vi "HE_state.vi"(6 "ZB":bool[](array[boolean])=[FALSE, FALSE], 7 "Alarm":bool[](array[boolean])=[FALSE, FALSE], 9 "XB":bool[](array[boolean])=[FALSE, FALSE, FALSE, FALSE, FALSE], 10 "Z_control":T5={"Z_HSw"=1, "Z_HSetState"=enum."on", "Z_ASetState"=enum."on", "Z_DSetState"=enum."on"}, 11 "HE1_state_in":refnum<class "HE_state.lvclass">) -> (1 "YB":bool[](array[boolean]), 2 "Z":T1={"Z_Source"=enum."local disabled", "Z_SetState"=enum."on", "Z_State"=enum."alarm", "Z_State_T"=0, "ZM_State"=enum."initialization", "ZM_State_T"=0, "ALR  L1"=FALSE, "ALR  L2"=FALSE, "HH_run"=0}, 3 "HE1_state_out":refnum<class "HE_state.lvclass">, 5 "ALR_ON":bool[](array[boolean]))   [LabVIEW 2019, in "Heating.lvlib" / "HE_state.lvclass"]
uses:
  HE_state.lvclass
  ctl/Z_control.ctl
  ctl/Z_State.ctl
  ctl/Z.ctl
  ctl/Z_source.ctl
  ctl/ZM_State.ctl
  HE_state.lvclass/HE_state.ctl
  ZM_state/HE_ZM_state.lvclass/HE_ZM_state.ctl
  Z_state/HE_Z_state.lvclass/HE_Z_state.ctl
  Sequence/State/State.lvclass/State.ctl
  Sequence/State/Read T (ms).vi
  Z_state/HE_Z_state.lvclass
  D:/my_projects/projects/Algorithms/Labview/19/Sequence/State/State.lvclass
  ZM_state/HE_ZM_state.lvclass
  Sequence/State/Step.vi
  Heating.lvlib
panel:
  # "Alarm_L1"
  # "Alarm_L2"
  # "Ki_XB01 contactor on"
  # "Ki_XB02 contactor off"
  # "XB24 local hand on"
  # "heating end"
  # "cooling end"
  # "Ki_ZB01 contactor on reg"
  # "Ki_ZB02 contactor off reg"
  # "TsStop"
  # "T_check"
  # "T_start_delay"
  # "T_heat_start"
  # "T_stop_delay"
  # "T_set_min"
  # "T_heat_stop"
  # "T_restart_delay"
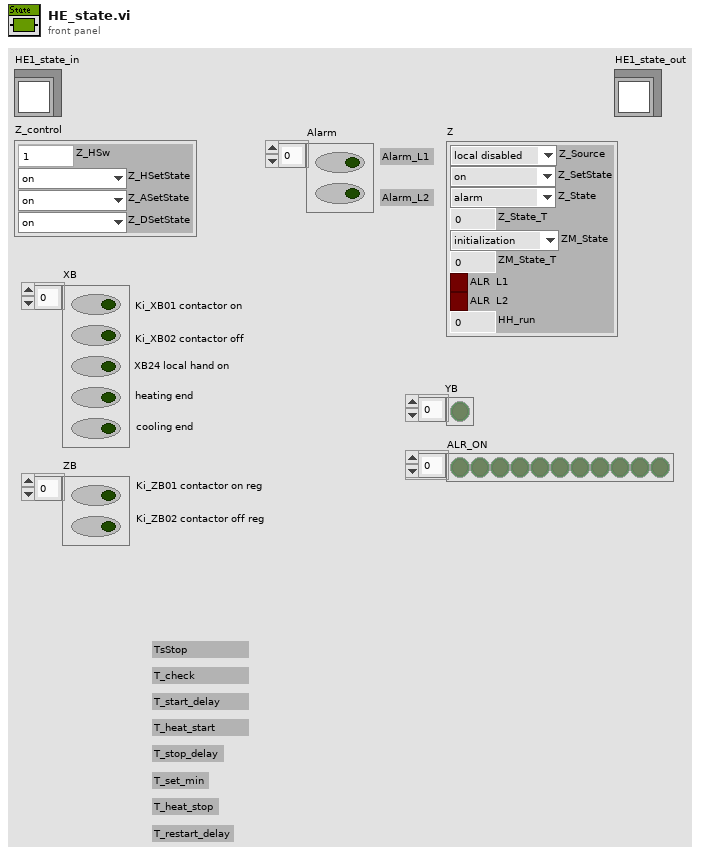
[diagram p1: front panel]
types:
  T1 = typedef "Heating.lvlib/Z.ctl" = cluster{"Z_Source":T2, "Z_SetState":T3, "Z_State":T3, "Z_State_T":u32, "ZM_State":T4, "ZM_State_T":u32, "ALR  L1":bool, "ALR  L2":bool, "HH_run":u64}
  T2 = typedef "Heating.lvlib/Z_source.ctl" = enum8{"initialize", "local disabled", "local hand", "hand", "auto", "dist"}
  T3 = typedef "Heating.lvlib/Z_State.ctl" = enum8{"initialization", "alarm", "disabled", "not ready", "stop ready", "reserv", "switched off", "reserv2", "switched on", "check", "on min", "decrease out", "on", "increase out", "on max"}
  T4 = typedef "Heating.lvlib/ZM_State.ctl" = enum8{"initialization", "stop", "start_cmd", "contactor_on_cmd", "heating", "on", "stop_cmd", "power_down", "contactor_off_cmd", "cooling", "restart_delay"}
  T5 = typedef "Heating.lvlib/Z_control.ctl" = cluster{"Z_HSw":u8, "Z_HSetState":T3, "Z_ASetState":T3, "Z_DSetState":T3}
  T6 = cluster{"Z_Source":T2, "Z_SetState":T3, "ZM_State":T4}
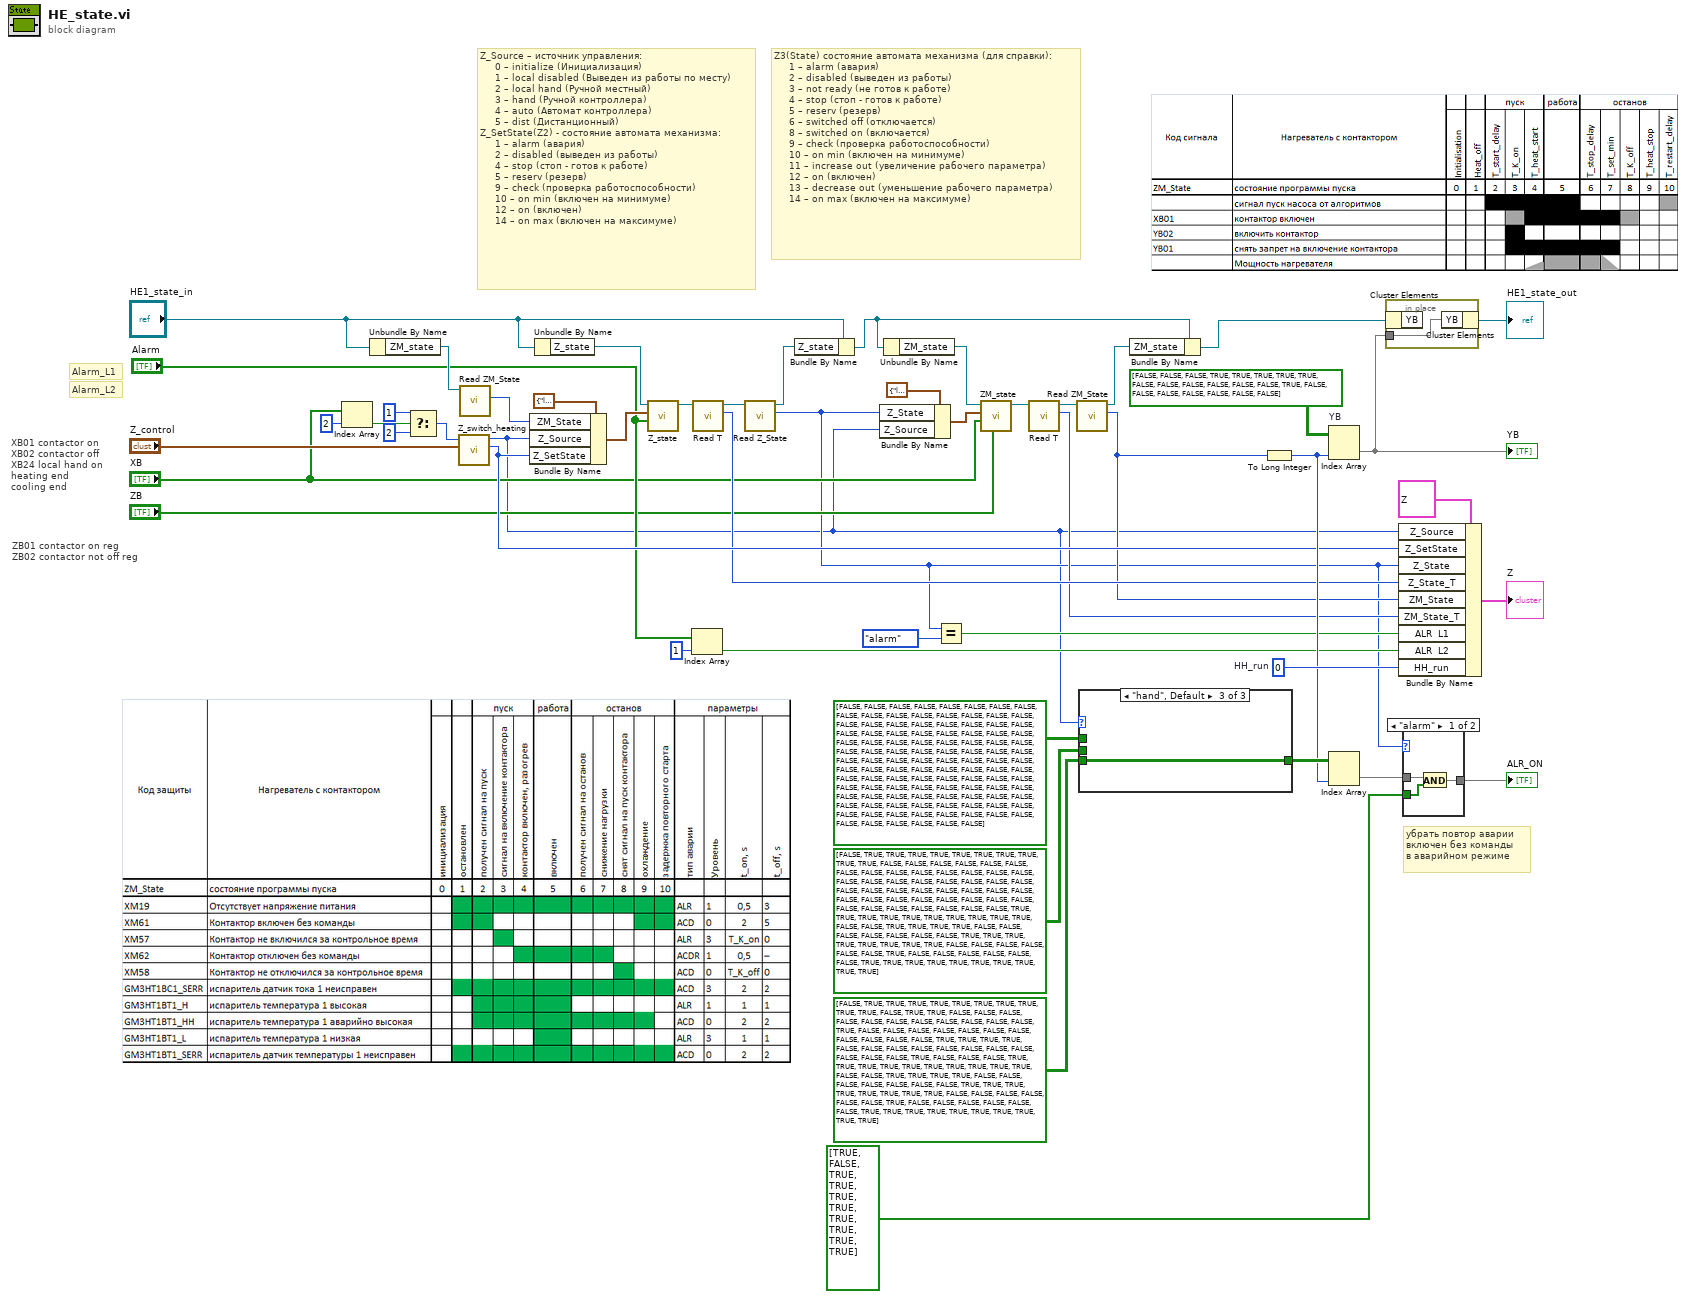
[diagram p0: block diagram]
diagram:
  w34 = 0  # HH_run
  # "Alarm_L2"
  # "Alarm_L1"
  # "ZB01 contactor on reg\nZB02 contactor not off reg"
  # "XB01 contactor on\nXB02 contactor off\nXB24 local hand on\nheating end\ncooling end"
  # "убрать повтор аварии\nвключен без команды\nв аварийном режиме"
  # "Z_Source – источник управления:\n     0 – initialize (Инициализация)\n     1 – local disabled (Выведен из работы по месту)\n     2 – local hand (Ручной местный)\n     3 – hand (Ручной контроллера)\n     4 – auto (Автомат контроллера)\n     5 – dist (Дистанционный)\nZ_SetState(Z2) - состояние автомата механизма:\n     1 – alarm (авария)\n     2 – disabled (выведен из работы)\n     4 – stop (стоп - готов к работе)\n     5 – reserv (резерв)\n     9 – check (проверка работоспособности)\n     10 – on min (включен на минимуме)\n     12 – on (включен)\n     14 – on max (включен на максимуме)"
  # "Z3(State) состояние автомата механизма (для справки):\n     1 – alarm (авария)\n     2 – disabled (выведен из работы)\n     3 – not ready (не готов к работе)\n     4 – stop (стоп - готов к работе)\n     5 – reserv (резерв)\n     6 – switched off (отключается)\n     8 – switched on (включается)\n     9 – check (проверка работоспособности)\n     10 – on min (включен на минимуме)\n     11 – increase out (увеличение рабочего параметра)\n     12 – on (включен)\n     13 – decrease out (уменьшение рабочего параметра)\n     14 – on max (включен на максимуме)"
  n1 = Index Array(array="XB", index=2) -> (element=w36:bool)
  n2 = Unbundle By Name("HE1_state_in") -> ("ZM_state"=w26:refnum<class "HE_ZM_state.lvclass">)
  n3 = Select(t=u8 1, s=w36, f=u8 2) -> (s? t:f=w44:u8)
  n4 = call "Z_switch_heating.vi"("Z"="Z_control", "Z_LSw"=w44) -> ("Z_SetState"=w27:T3, "Z_Source"=w6:T2)  [unwired: 8 in]
  n5 = call "Read ZM_State.vi"("HE_ZM_state in"=w26) -> ("ZM_State"=w25:T4)  [unwired: 9 in, 1 out]
  n6 = Bundle By Name(cluster=T6 {"Z_Source"=enum."local disabled", "Z_SetState"=enum."alarm", "ZM_State"=enum."initialization"} ("Z_In"), "ZM_State"=w25, "Z_Source"=w6, "Z_SetState"=w27) -> (w24:T6)
  n7 = Unbundle By Name("HE1_state_in") -> ("Z_state"=w23:refnum<class "HE_Z_state.lvclass">)
  n8 = call "Z_state.vi"("Alarm"="Alarm", "Z_In"=w24, "HE1_Z_state in"=w23) -> ("HE1_Z_state out"=w21:refnum<class "HE_Z_state.lvclass">)  [unwired: 8 in]
  n9 = Index Array(array="Alarm", index=1) -> (element=w29:bool)
  n10 = call "Read T.vi"("HE1_Z_state in"=w21) -> ("T (ms)"=w19:u32, "HE1_Z_state out"=w20:refnum<class "HE_Z_state.lvclass">)  [unwired: 9 in]
  n11 = call "Read Z_State.vi"("HE1_Z_state in"=w20) -> ("Z_State_heating"=w8:T3, "HE1_Z_state out"=w17:refnum<class "HE_Z_state.lvclass">)  [unwired: 9 in]
  n12 = Bundle By Name(cluster="HE1_state_in", "Z_state"=w17) -> (w4:refnum<class "HE_state.lvclass">)
  n13 = Bundle By Name(cluster=cluster{"Z_Source":T2, "Z_State":T3} {"Z_Source"=enum."local disabled", "Z_State"=enum."alarm"} ("Z_In"), "Z_State"=w8, "Z_Source"=w6) -> (w7:cluster{"Z_Source":T2, "Z_State":T3})
  n14 = Unbundle By Name(w4) -> ("ZM_state"=w16:refnum<class "HE_ZM_state.lvclass">)
  n15 = Equal?(x=w8, y=Z_State."alarm") -> (x = y?=w31:bool)
  n16 = call "ZM_state.vi"("ZB"="ZB", "XB"="XB", "Z_In"=w7, "ZM_state in"=w16) -> ("ZM_state out"=w15:refnum<class "HE_ZM_state.lvclass">)  [unwired: 7 in]
  n17 = call "Read T.vi"("valve_VCH_ZM_state in"=w15) -> ("T (ms)"=w12:u32, "valve_VCH_ZM_state out"=w14:refnum<class "HE_ZM_state.lvclass">)  [unwired: 9 in]
  n18 = call "Read ZM_State.vi"("HE_ZM_state in"=w14) -> ("ZM_State"=w13:T4, "HE_ZM_state out"=w5:refnum<class "HE_ZM_state.lvclass">)  [unwired: 9 in]
  n19 = case shown="\"hand\", Default" w6 {
    tunnel: bool[][] [[FALSE, FALSE, FALSE, FALSE, FALSE, FALSE, FALSE, FALSE, FALSE, FALSE, FALSE], [FALSE, FALSE, FALSE, FALSE, FALSE, FALSE, FALSE, FALSE, FALSE, FALSE, FALSE], [FALSE, FALSE, FALSE, FALSE, FALSE, FALSE, FALSE, FALSE, FALSE, FALSE, FALSE], [FALSE, FALSE, FALSE, FALSE, FALSE, FALSE, FALSE, FALSE, FALSE, FALSE, FALSE], [FALSE, FALSE, FALSE, FALSE, FALSE, FALSE, FALSE, FALSE, FALSE, FALSE, FALSE], [FALSE, FALSE, FALSE, FALSE, FALSE, FALSE, FALSE, FALSE, FALSE, FALSE, FALSE], [FALSE, FALSE, FALSE, FALSE, FALSE, FALSE, FALSE, FALSE, FALSE, FALSE, FALSE], [FALSE, FALSE, FALSE, FALSE, FALSE, FALSE, FALSE, FALSE, FALSE, FALSE, FALSE], [FALSE, FALSE, FALSE, FALSE, FALSE, FALSE, FALSE, FALSE, FALSE, FALSE, FALSE], [FALSE, FALSE, FALSE, FALSE, FALSE, FALSE, FALSE, FALSE, FALSE, FALSE, FALSE]] -> [w51 _ _]
    tunnel: bool[][] [[FALSE, TRUE, TRUE, TRUE, TRUE, TRUE, TRUE, TRUE, TRUE, TRUE, TRUE], [FALSE, FALSE, FALSE, FALSE, FALSE, FALSE, FALSE, FALSE, FALSE, FALSE, FALSE], [FALSE, FALSE, FALSE, FALSE, FALSE, FALSE, FALSE, FALSE, FALSE, FALSE, FALSE], [FALSE, FALSE, FALSE, FALSE, FALSE, FALSE, FALSE, FALSE, FALSE, FALSE, FALSE], [FALSE, FALSE, FALSE, FALSE, FALSE, FALSE, FALSE, FALSE, FALSE, FALSE, FALSE], [FALSE, TRUE, TRUE, TRUE, TRUE, TRUE, TRUE, TRUE, TRUE, TRUE, TRUE], [FALSE, FALSE, TRUE, TRUE, TRUE, TRUE, FALSE, FALSE, FALSE, FALSE, FALSE], [FALSE, FALSE, TRUE, TRUE, TRUE, TRUE, TRUE, TRUE, TRUE, TRUE, FALSE], [FALSE, FALSE, FALSE, FALSE, FALSE, TRUE, FALSE, FALSE, FALSE, FALSE, FALSE], [FALSE, TRUE, TRUE, TRUE, TRUE, TRUE, TRUE, TRUE, TRUE, TRUE, TRUE]] -> [_ w52 _]
    tunnel: bool[][] [[FALSE, TRUE, TRUE, TRUE, TRUE, TRUE, TRUE, TRUE, TRUE, TRUE, TRUE], [FALSE, TRUE, TRUE, FALSE, FALSE, FALSE, FALSE, FALSE, FALSE, FALSE, FALSE], [FALSE, FALSE, FALSE, TRUE, FALSE, FALSE, FALSE, FALSE, FALSE, FALSE, FALSE], [FALSE, FALSE, FALSE, FALSE, TRUE, TRUE, TRUE, TRUE, FALSE, FALSE, FALSE], [FALSE, FALSE, FALSE, FALSE, FALSE, FALSE, FALSE, FALSE, TRUE, FALSE, FALSE], [FALSE, TRUE, TRUE, TRUE, TRUE, TRUE, TRUE, TRUE, TRUE, TRUE, TRUE], [FALSE, FALSE, TRUE, TRUE, TRUE, TRUE, FALSE, FALSE, FALSE, FALSE, FALSE], [FALSE, FALSE, TRUE, TRUE, TRUE, TRUE, TRUE, TRUE, TRUE, TRUE, FALSE], [FALSE, FALSE, FALSE, FALSE, FALSE, TRUE, FALSE, FALSE, FALSE, FALSE, FALSE], [FALSE, TRUE, TRUE, TRUE, TRUE, TRUE, TRUE, TRUE, TRUE, TRUE, TRUE]] -> [_ _ w53]
    tunnel: [w51 w52 w53] -> w48
    frame "initialize", "local disabled" {
    }
    frame "local hand" {
    }
    frame "hand", Default {
    }
  }
  n20 = Bundle By Name(cluster=w4, "ZM_state"=w5) -> (w3:refnum<class "HE_state.lvclass">)
  n21 = To Long Integer(number=w13) -> (32bit integer=w33:i32)
  n22 = Index Array "YB"(array=bool[][] [[FALSE, FALSE, FALSE, TRUE, TRUE, TRUE, TRUE, TRUE, FALSE, FALSE, FALSE], [FALSE, FALSE, FALSE, TRUE, FALSE, FALSE, FALSE, FALSE, FALSE, FALSE, FALSE]], index (col)=w33) -> (element=w2:bool[])  [unwired: 1 in]
  "YB" <- w2
  n23 = Index Array(array=w48, index (col)=w33) -> (element=w47:bool[])  [unwired: 1 in]
  n24 = in-place {
    in-place-border: w2 -> [w54]
    n25 = in-place-cluster #1(w3) -> ()  [unwired: 1 out]
    n26 = in-place-cluster #1("YB"=w54) -> (→"HE1_state_out":refnum<class "HE_state.lvclass">)
  }
  n27 = Bundle By Name(cluster=T1 {"Z_Source"=enum."local disabled", "Z_SetState"=enum."on", "Z_State"=enum."alarm", "Z_State_T"=0, "ZM_State"=enum."initialization", "ZM_State_T"=0, "ALR  L1"=FALSE, "ALR  L2"=FALSE, "HH_run"=0} ("Z"), "Z_Source"=w6, "Z_SetState"=w27, "Z_State"=w8, "Z_State_T"=w19, "ZM_State"=w13, "ZM_State_T"=w12, "ALR  L1"=w31, "ALR  L2"=w29, "HH_run"=w34) -> (→"Z":T1)
  n28 = case shown="\"alarm\"" w8 {
    tunnel: bool[] [TRUE, FALSE, TRUE, TRUE, TRUE, TRUE, TRUE, TRUE, TRUE, TRUE] -> [w56 _]
    tunnel: w47 -> [w57 w58]
    tunnel: [w55 w58] -> w46
    frame "alarm" {
      n29 = And(x=w57, y=w56) -> (x .and. y?=w55:bool[])
    }
    frame "disabled", Default {
    }
  }
  "ALR_ON" <- w46
